vi "Data_Display_global_test.vi"() -> ()   [LabVIEW 2018]
uses:
  Monitors/Utility/Monitor Communication/SR830/SR830-Cluster.ctl
  Monitors/Utility/Monitor Communication/S16/16T-Cluster.ctl
panel:
  out "Magnetic Field SC":dbl
  in  "16 T Cluster":T1={"Clamp"=FALSE, "Switch Heater"=FALSE, "Go to Zero"=FALSE, "Go to set"=FALSE, "Go to Hold"=FALSE, "Clamped"=FALSE, "Quenched"=FALSE, "Rate limit"=FALSE, "Persistent"=FALSE, "Hold"=FALSE, "Set"=FALSE, "Zero"=FALSE, "Magnet (T)"=0.0, "Leads (T)"=0.0, "Magnet T (K)"=3.4572, "Switch"=FALSE, "Setpoint (T)"=3.4572, "Rate (T/min)"=0.0, "Select"=FALSE, "Sweeping"=FALSE} caption="16 T Magnet control" {"Rate (T/min)" format="%6_5f"; "Setpoint (T)" format="%6_5f"; "Magnet T (K)" format="%#4_5f"; "Leads (T)" format="%6_5f"}
  out "SR830-Running 3":bool
  out "SR830-Running 2":bool
  out "SR830-Running":bool
  out "SR830-3":T2={"Lockin 1"=[], "X1-Display"=0.0, "Y1-Display"=0.0, "X1 Percent"=0.0, "X1 Overload"=FALSE, "Y1 Overload"=FALSE, "Unit X1"="nV", "Unit X2"="nV", "Unit X2a"="nV", "Unit X1a"="nV", "Sensitivity Setpoint"=26, "X1 Percent 2"=0.0, "Y1"=0.0, "X1"=0.0, "Preamp OVL"=FALSE} {"X1 Percent 2" scale=0.0..1.0; "Sensitivity Setpoint" items=["2 nV", "5 nV", "10 nV", "20 nV", "50 nV", "100 nV", "200 nV", "500 nV", "1 µV", "2 µV", "5 µV", "10 µV", "20 µV", "50 µV", "100 µV", "200 µV", "500 µV", "1 mV", "2 mV", "5 mV", "10 mV", "20 mV", "50 mV", "100 mV", "200 mV", "500 mV", "1 V", ""]; "X1 Percent" scale=0.0..1.0; "X1-Display" format="%#4_5f"}
  out "SR830-2":T2={"Lockin 1"=[], "X1-Display"=0.0, "Y1-Display"=0.0, "X1 Percent"=0.0, "X1 Overload"=FALSE, "Y1 Overload"=FALSE, "Unit X1"="nV", "Unit X2"="nV", "Unit X2a"="nV", "Unit X1a"="nV", "Sensitivity Setpoint"=26, "X1 Percent 2"=0.0, "Y1"=0.0, "X1"=0.0, "Preamp OVL"=FALSE} {"X1 Percent 2" scale=0.0..1.0; "Sensitivity Setpoint" items=["2 nV", "5 nV", "10 nV", "20 nV", "50 nV", "100 nV", "200 nV", "500 nV", "1 µV", "2 µV", "5 µV", "10 µV", "20 µV", "50 µV", "100 µV", "200 µV", "500 µV", "1 mV", "2 mV", "5 mV", "10 mV", "20 mV", "50 mV", "100 mV", "200 mV", "500 mV", "1 V", ""]; "X1 Percent" scale=0.0..1.0; "X1-Display" format="%#4_5f"}
  out "Error":bool
  out "Critical Error":bool
  in  "Error String":string
  out "SR830-1":T2={"Lockin 1"=[], "X1-Display"=0.0, "Y1-Display"=0.0, "X1 Percent"=0.0, "X1 Overload"=FALSE, "Y1 Overload"=FALSE, "Unit X1"="nV", "Unit X2"="nV", "Unit X2a"="nV", "Unit X1a"="nV", "Sensitivity Setpoint"=26, "X1 Percent 2"=0.0, "Y1"=0.0, "X1"=0.0, "Preamp OVL"=FALSE} {"X1 Percent 2" scale=0.0..1.0; "Sensitivity Setpoint" items=["2 nV", "5 nV", "10 nV", "20 nV", "50 nV", "100 nV", "200 nV", "500 nV", "1 µV", "2 µV", "5 µV", "10 µV", "20 µV", "50 µV", "100 µV", "200 µV", "500 µV", "1 mV", "2 mV", "5 mV", "10 mV", "20 mV", "50 mV", "100 mV", "200 mV", "500 mV", "1 V", ""]; "X1 Percent" scale=0.0..1.0; "X1-Display" format="%#4_5f"}
  out "AVS R7":dbl
  out "AVS R6":dbl
  out "AVS R5":dbl
  out "LS370 auto excitation":bool
  out "LS370 setpoint":dbl
  out "Magnet Degaussing finished":bool
  out "VCM amplitude":dbl
  out "VCM frequency":dbl
  out "LS370 heater power(W)":dbl
  out "Stop Monitors":bool
  out "AVS Temperature Monitor active":bool
  out "AVS Resitance Monitor active":bool
  out "LS370 T2":dbl
  out "LS370 R2":dbl
  out "Degauss":bool
  out "Wait":bool
  out "Tstep":bool
  out "LS370 T5":dbl
  out "LS370 T4":dbl
  out "LS370 T3":dbl
  out "LS370 T1":dbl
  out "LS370 R5":dbl
  out "LS370 R4":dbl
  out "LS370 R3":dbl
  out "LS370 R1":dbl
  out "Const":bool
  out "Bstep":bool
  out "Script succeeded":bool
  out "AVS Resistance":dbl
  out "SR830#3 Ch2":dbl
  out "SR830#3 Ch1":dbl
  out "SR850 Ch2":dbl
  out "SR850 Ch1":dbl
  out "Step width":dbl
  out "PE7265 Ch2":dbl
  out "PE7265 Ch1":dbl
  out "Sample Temperature Lakeshore 340":dbl
  out "current I setpoint":dbl
  out "Voltage":dbl
  out "Resistance":dbl
  out "Current":dbl
  out "needle valve (%)":dbl
  out "LS370 readout power(W)":dbl
  out "CC running time":dbl
  out "waiting time":dbl
  out "current number of steps":i32
  out "current field setpoint":dbl
  out "Bramp":bool
  out "B_init reached":bool
  out "Tramp":bool
  out "T_init reached":bool
  out "SR830#2 Ch2":dbl
  out "SR830#2 Ch1":dbl
  out "SR830#1 Ch2":dbl
  out "SR830#1 Ch1":dbl
  out "Magnetic Field":dbl
  out "LS370 Temperature":dbl
  out "AVS Temperature":dbl
  out "Init/SC Selector":bool
  # "General Settings"
  # "Temperature Reading"
  # "Lock-In Reading"
  # "Sequence communictions"
  # "VCM data"
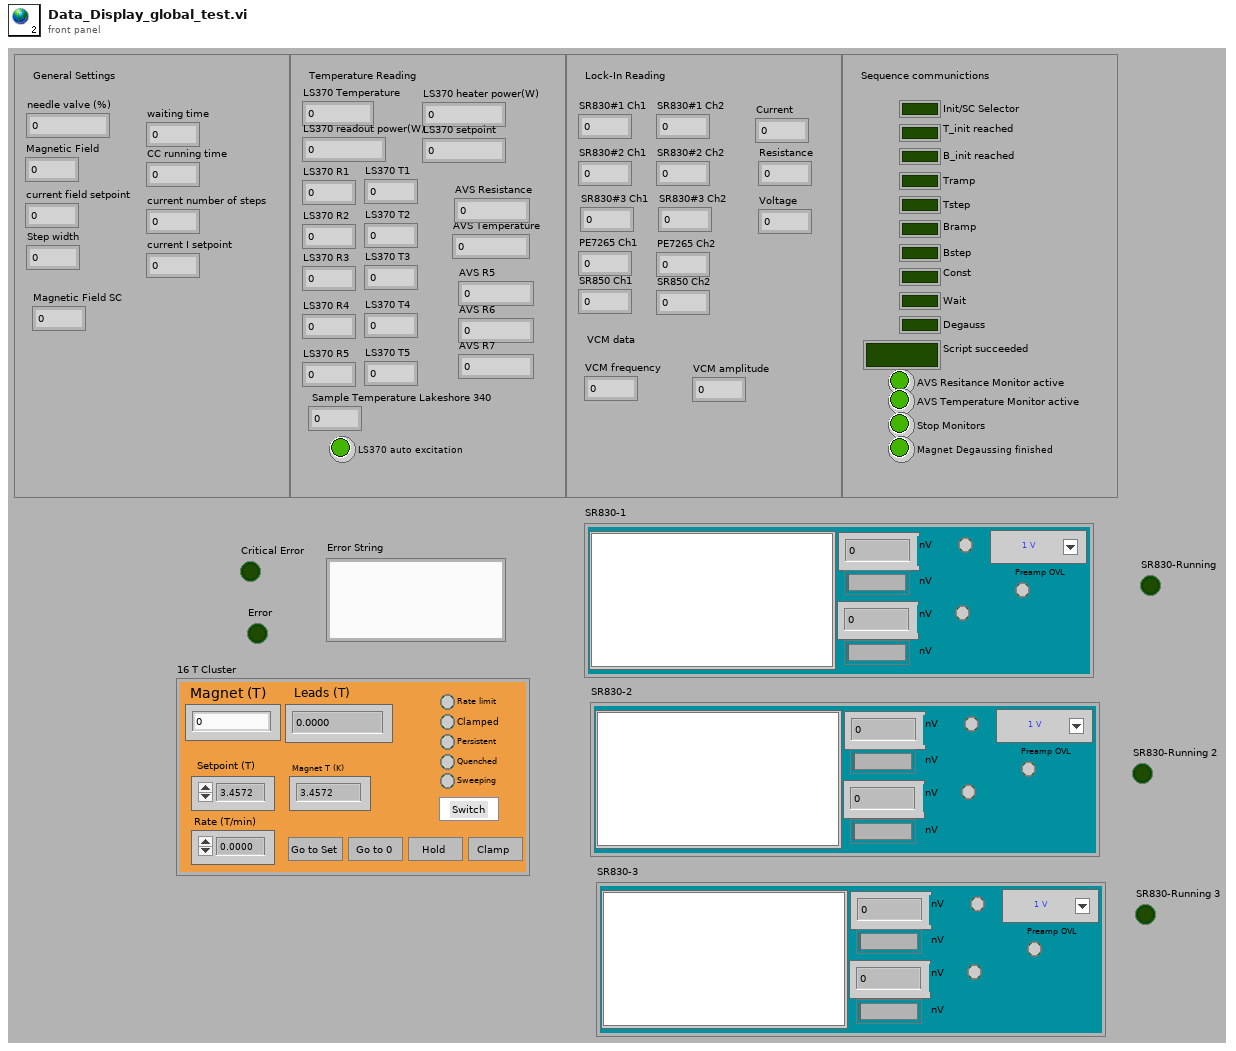
[diagram p1: front panel]
types:
  T1 = typedef "16T-Cluster.ctl" = cluster{"Clamp":bool, "Switch Heater":bool, "Go to Zero":bool, "Go to set":bool, "Go to Hold":bool, "Clamped":bool, "Quenched":bool, "Rate limit":bool, "Persistent":bool, "Hold":bool, "Set":bool, "Zero":bool, "Magnet (T)":dbl, "Leads (T)":dbl, "Magnet T (K)":dbl, "Switch":bool, "Setpoint (T)":dbl, "Rate (T/min)":dbl, "Select":bool, "Sweeping":bool}
  T2 = typedef "SR830-Cluster.ctl" = cluster{"Lockin 1":dbl[][], "X1-Display":dbl, "Y1-Display":dbl, "X1 Percent":dbl, "X1 Overload":bool, "Y1 Overload":bool, "Unit X1":string, "Unit X2":string, "Unit X2a":string, "Unit X1a":string, "Sensitivity Setpoint":i16, "X1 Percent 2":dbl, "Y1":dbl, "X1":dbl, "Preamp OVL":bool}
diagram:
